vi "Drive Check for New Command.vi"(9 "input cluster":T7, 10 "Wait time (ms)":dbl, 11 "Finished?":bool) -> (0 "Completion":T5, 1 "Subsystem Name":string, 2 "Current Command":T1, 3 "Initial Trace String":string, 4 "Next Command":T7)   [LabVIEW 2023]
doc: "This VI is called for each controller loop iteration. It checks for new commands, updates timing data, and upon completion, notifies and waiting commands."
uses:
  Drive Setpoints.ctl
  Drive Operations.ctl
  swerve/Type Definitions/Data/Robot Velocities.ctl
  <vilib>/Rock Robotics/WPI/Framework/Command Status Info.ctl
  <vilib>/Rock Robotics/WPI/Framework/Completion Status.ctl
  <vilib>/Rock Robotics/WPI/Framework/Completion Notifier.ctl
  Drive Published Globals.vi
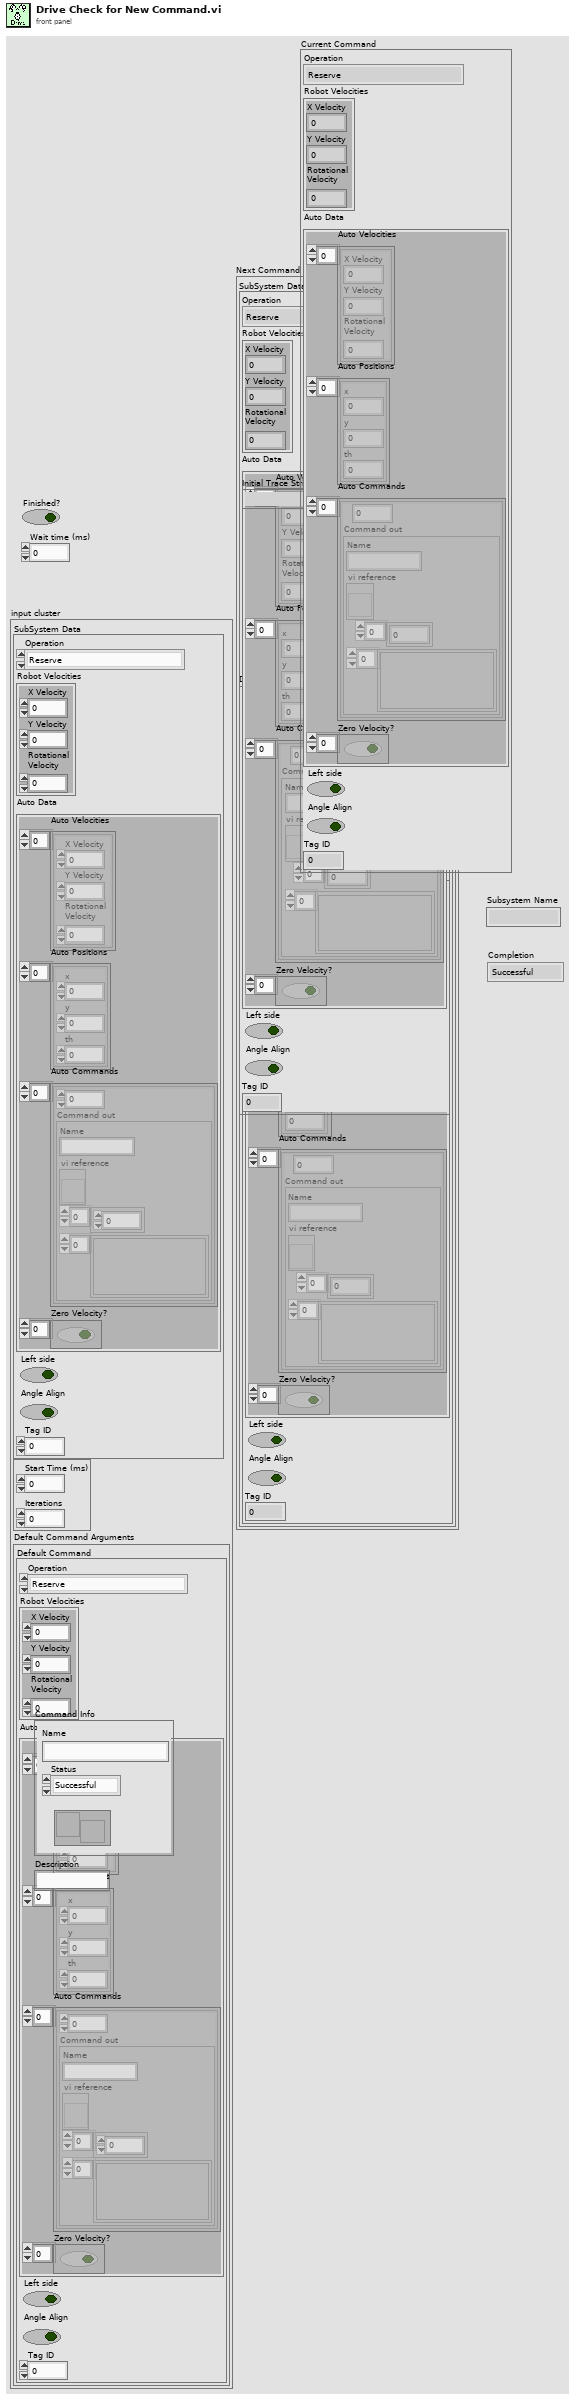
[diagram p1: front panel]
types:
  T1 = typedef "Drive Setpoints.ctl" = cluster{"Operation":T2, "Robot Velocities":T3, "Auto Data":cluster{"Auto Velocities":T3[], "Auto Positions":cluster{"x":dbl, "y":dbl, "th":dbl}[], "Auto Commands":cluster{dbl, "Command out":cluster{"Name":string, "vi reference":refnum<vi>, i32[], variant[]}}[], "Zero Velocity?":bool[]}, "Left side":bool, "Angle Align":bool, "Tag ID":i32}
  T2 = typedef "Drive Operations.ctl" = enum16{"Reserve", "Read Current", "Immediate", "Calibrate", "Reef Align", "Auto", "Old Reef Align"}
  T3 = typedef "Robot Velocities.ctl" = cluster{"X Velocity":dbl, "Y Velocity":dbl, "Rotational \nVelocity":dbl}
  T4 = typedef "Command Status Info.ctl" = cluster{"Name":string, "Status":T5, "notifier out":T6}
  T5 = typedef "Completion Status.ctl" = enum16{"Successful", "Aborted", "Incomplete"}
  T6 = typedef "Completion Notifier.ctl" = refnum<notifier>
  T7 = cluster{"SubSystem Data":T1, cluster{"Start Time (ms)":u32, "Iterations":i32}, "Default Command Arguments":cluster{"Command Info":T4, "Description":string, "Default Command":T1, "queue out":refnum<queue>, "Subsystem Name":string}}
  T8 = cluster{"Command Info":T4, "Description":string, "Default Command":T1, "queue out":refnum<queue>, "Subsystem Name":string}
  T9 = cluster{"Default Command":T1, "Command Info":T4, "Description":string}
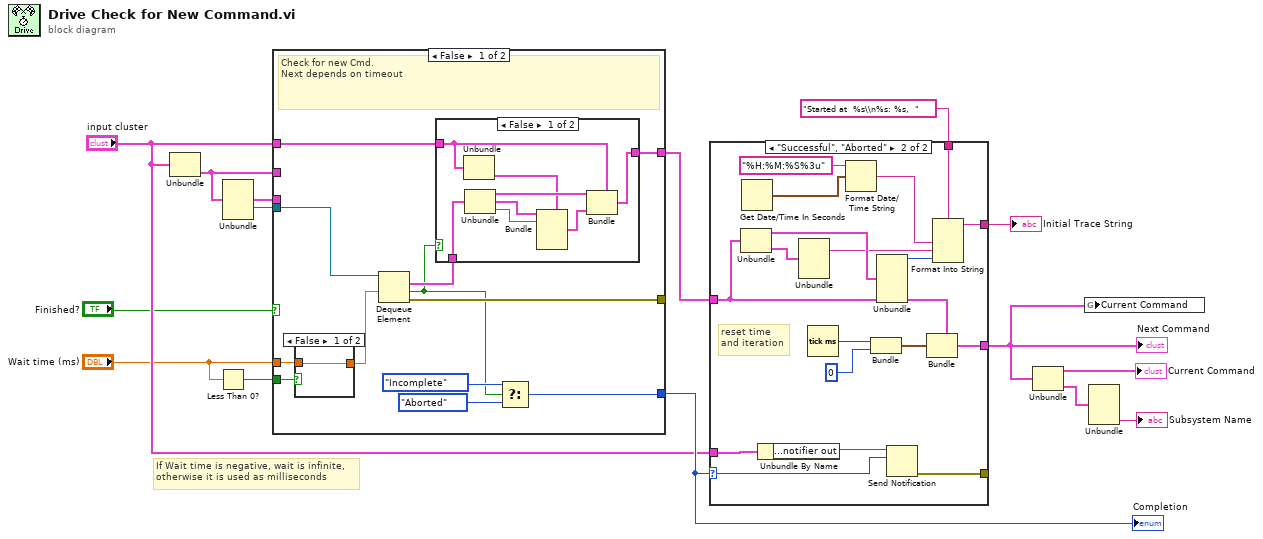
[diagram p0: block diagram]
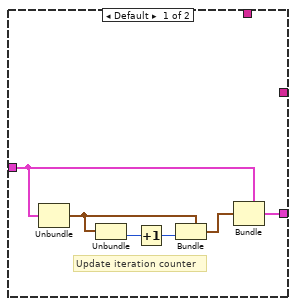
[diagram p2: hidden frame]
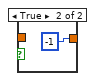
[diagram p4: hidden frame]
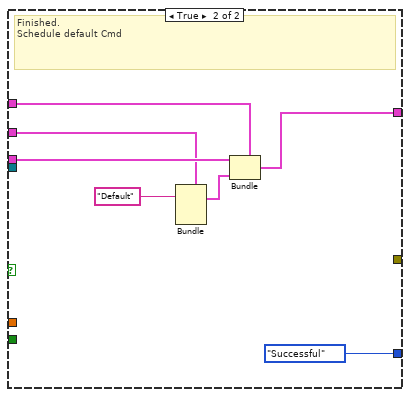
[diagram p5: hidden frame]
diagram:
  # "If Wait time is negative, wait is infinite,\notherwise it is used as milliseconds"
  n1 = Unbundle("input cluster") -> ("Default Command Arguments"=w4:T8)  [unwired: 2 out]
  n2 = Less Than 0?(x="Wait time (ms)") -> (x < 0?=w2:bool)
  n3 = Unbundle(w4) -> ("Default Command"=w7:T1, "queue out"=w8:refnum<queue>)  [unwired: 3 out]
  n4 = case shown="False" "Finished?" {
    tunnel: [w23 w44] -> w11
    tunnel: w2 -> [w17 _]
    tunnel: [w27 Completion_Status."Successful"] -> w15
    tunnel: [w20 _] -> _
    tunnel: w8 -> [w22 _]
    tunnel: "input cluster" -> [w24 w43]
    tunnel: w7 -> [_ w42]
    tunnel: w4 -> [_ w40]
    tunnel: "Wait time (ms)" -> [w16 _]
    frame False {
      # "Check for new Cmd.\nNext depends on timeout"
      n5 = case shown="False" w17 {
        tunnel: [w37 -1] -> w21
        tunnel: w16 -> [w37 _]
        frame False {
        }
        frame True {
        }
      }
      n6 = Dequeue Element(queue=w22, timeout in ms (-1)=w21) -> (element=w19:T9, timed out?=w18:bool, error out=w20:errorcluster)  [unwired: 1 in, 1 out]
      n7 = case shown="False" w18 {
        tunnel: w19 -> [w35 _]
        tunnel: w24 -> [w32 w36]
        tunnel: [w28 w36] -> w23
        frame False {
          n8 = Unbundle(w32) -> ("Default Command Arguments"=w31:T8)  [unwired: 2 out]
          n9 = Unbundle(w35) -> ("Default Command"=w34:T1, "Command Info"=w29:T4, "Description"=w30:string)
          n10 = Bundle(cluster=w31, "Command Info"=w29, "Description"=w30) -> (w33:T8)  [unwired: 3 in]
          n11 = Bundle(cluster=w32, "SubSystem Data"=w34, "Default Command Arguments"=w33) -> (w28:T7)  [unwired: 1 in]
        }
        frame True {
        }
      }
      n12 = Select(t=Completion_Status."Incomplete", s=w18, f=Completion_Status."Aborted") -> (s? t:f=w27:T5)
    }
    frame True {
      # "Finished.\nSchedule default Cmd"
      n13 = Bundle(cluster=w40, "Description"="Default") -> (w41:T8)  [unwired: 4 in]
      n14 = Bundle(cluster=w43, "SubSystem Data"=w42, "Default Command Arguments"=w41) -> (w44:T7)  [unwired: 1 in]
    }
  }
  "Completion" <- w15
  n15 = case shown="\"Successful\", \"Aborted\"" w15 {
    selector: w15 -> [_ w69]
    tunnel: "input cluster" -> [_ w57]
    tunnel: "Started at  %s\\n%s: %s,  " ("format string") -> [_ w66]
    tunnel: [_ w65] -> w13
    tunnel: w11 -> [w48 w58]
    tunnel: [w49 w62] -> w3
    tunnel: [_ w59] -> _
    frame Default {
      # "Update iteration counter"
      n16 = Unbundle(w48) -> (w47:cluster{"Start Time (ms)":u32, "Iterations":i32})  [unwired: 2 out]
      n17 = Unbundle(w47) -> ("Iterations"=w50:i32)  [unwired: 1 out]
      n18 = Increment(x=w50) -> (x+1=w51:i32)
      n19 = Bundle(cluster=w47, "Iterations"=w51) -> (w46:cluster{"Start Time (ms)":u32, "Iterations":i32})  [unwired: 1 in]
      n20 = Bundle(cluster=w48, w46) -> (w49:T7)  [unwired: 2 in]
    }
    frame "Successful", "Aborted" {
      # "reset time\nand iteration"
      n21 = Unbundle(w58) -> ("SubSystem Data"=w64:T1, "Default Command Arguments"=w60:T8)  [unwired: 1 out]
      n22 = Get Date/Time In Seconds() -> (seconds since 1Jan1904=w53:timestamp)
      n23 = Unbundle By Name(w57) -> ("Default Command Arguments.Command Info.notifier out"=w68:T6)
      n24 = Unbundle(w60) -> ("Description"=w55:string)  [unwired: 4 out]
      n25 = Tick Count (ms)() -> (millisecond timer value=w56:u32)
      n26 = Format Date/Time String(time format string (%c)="%H:%M:%S%3u", seconds (now)=w53) -> (date/time string=w52:string)  [unwired: 1 in]
      n27 = Bundle("millisecond timer value"=w56, 0) -> (w61:cluster{"millisecond timer value":u32, i32})  [unwired: 1 in]
      n28 = Unbundle(w64) -> ("Operation"=w67:T2)  [unwired: 5 out]
      n29 = Send Notification(notification=w69, notifier=w68) -> (error out=w59:errorcluster)  [unwired: 1 in, 1 out]
      n30 = Bundle(cluster=w58, w61) -> (w62:T7)  [unwired: 2 in]
      n31 = Format Into String(format string=w66, w52, w55, w67) -> (resulting string=w65:string)  [unwired: 2 in, 1 out]
    }
  }
  "Next Command" <- w3
  "Initial Trace String" <- w13
  n32 = Unbundle(w3) -> ("SubSystem Data"=→"Current Command":T1, "Default Command Arguments"=w6:T8)  [unwired: 1 out]
  n33 = global write "Drive Published Globals.vi" "Current Command"(w3) -> ()
  n34 = Unbundle(w6) -> ("Subsystem Name"=→"Subsystem Name":string)  [unwired: 4 out]
